vi "Convert State For Save 1.vi"(2 "Container State":T1, 3 "Display State":T2) -> (1 "Display State To Save":variant)   [LabVIEW 2014, in "GCode_Xcontrol.xctl"]
uses:
  GCode_Xcontrol.xctl
  State 1.ctl
  <vilib>/_xctls/Container State.ctl
  <vilib>/_xctls/XControlSupport.lvlib
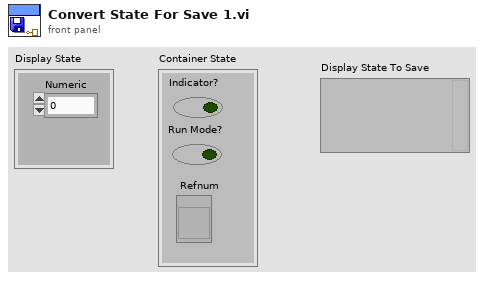
[diagram p1: front panel]
types:
  T1 = typedef "XControlSupport.lvlib/Container State.ctl" = cluster{"Indicator?":bool, "Run Mode?":bool, " Refnum":refnum<vi>}
  T2 = typedef "GCode_Xcontrol.xctl/State 1.ctl" = cluster{"Numeric":dbl}
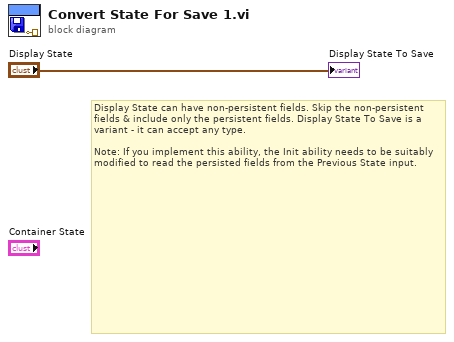
[diagram p0: block diagram]
diagram:
  # "Display State can have non-persistent fields. Skip the non-persistent fields & include only the persistent fields. Display State To Save is a variant - it can accept any type.\n\nNote: If you implement this ability, the Init ability needs to be suitably modified to read the persisted fields from the Previous State input."
  "Display State To Save" <- "Display State"
